vi "ELait03_CriticalValue.vi"(11 "DriverConnect":T1) -> (3 "output string":string)   [LabVIEW 2018]
uses:
  MOKO_LabViewLibrary/MokoLowLevel/MokoLowLovelControl/MLLC_ConnectCluster.ctl
  MOKO_LabViewLibrary/MokoLowLevel/MokoLowLovelControl/MLLC_InterfaceType.ctl
  MOKO_LabViewLibrary/MokoLowLevel/MokoLowLovelControl/MLLC_OpenedSession.ctl
  MOKO_LabViewLibrary/MokoLowLevel/MokoLowLovelControl/MLLC_InterfaceSettings.ctl
  MOKO_LabViewLibrary/MokoLowLevel/MokoLowLovelControl/MLLC_InterfaceKind.ctl
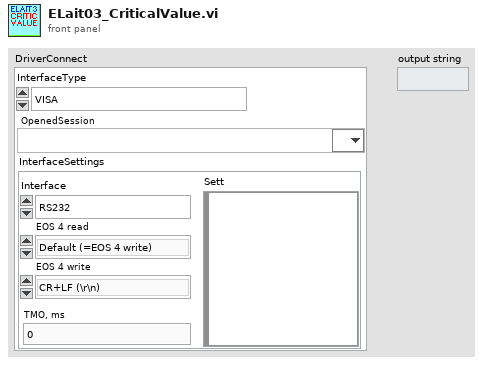
[diagram p1: front panel]
types:
  T1 = typedef "MLLC_ConnectCluster.ctl" = cluster{"InterfaceType":T2, "OpenedSession":T3, "InterfaceSettings":T4}
  T2 = typedef "MLLC_InterfaceType.ctl" = enum16{"VISA", "Prologix USB-GPIB"}
  T3 = typedef "MLLC_OpenedSession.ctl" = refnum<visa-resource-name>
  T4 = typedef "MLLC_InterfaceSettings.ctl" = cluster{"Interface":T5, "EOS 4 read":enum16{"Default (=EOS 4 write)", "CR (\\r)", "LF (\\n)", "None"}, "EOS 4 write":enum16{"CR+LF (\\r\\n)", "CR (\\r)", "LF (\\n)", "None"}, "TMO, ms":i32, "Sett":variant}
  T5 = typedef "MLLC_InterfaceKind.ctl" = enum16{"RS232", "GPIB", "USB", "Ethernet", "another"}
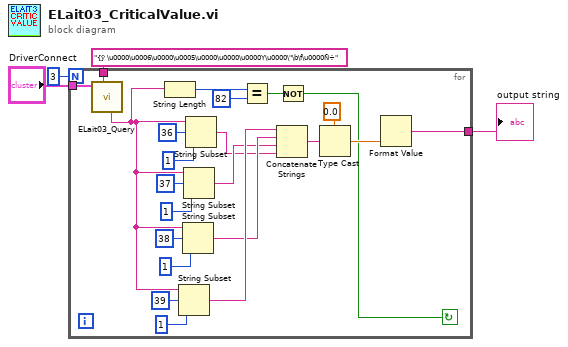
[diagram p0: block diagram]
diagram:
  n1 = for {
    N: 3 -> [_]
    tunnel: "DriverConnect" -> [w12]
    tunnel: "{ÿ \u0000\u0006\u0000\u0005\u0000\u0000\u0000Y\u0000\"\b\f\u0000Ñ÷" -> [w11]
    tunnel: [w10] -> w3
    stop <- w5 continue-if-true
    n2 = call "ELait03_Query.vi"("String"=w11, "DriverConnect in"=w12) -> ("String from device out"=w9:string)  [unwired: 7 in, 2 out]
    n3 = String Length(string=w9) -> (length=w8:i32)
    n4 = String Subset(string=w9, offset (0)=39, length (rest)=1 ("length (rest)")) -> (substring=w17:string)
    n5 = String Subset(string=w9, offset (0)=38, length (rest)=1 ("length (rest)")) -> (substring=w16:string)
    n6 = String Subset(string=w9, offset (0)=37, length (rest)=1 ("length (rest)")) -> (substring=w15:string)
    n7 = String Subset(string=w9, offset (0)=36, length (rest)=1 ("length (rest)")) -> (substring=w14:string)
    n8 = Equal?(x=w8, y=82) -> (x = y?=w6:bool)
    n9 = Concatenate Strings(w17, w16, w15, w14) -> (w13:string)
    n10 = Not(x=w6) -> (.not. x?=w5:bool)
    n11 = Type Cast(type=sgl 0.0, x=w13) -> (*(type *) &x=w18:sgl)
    n12 = Format Value(value (0)=w18) -> (output string=w10:string)  [unwired: 2 in]
  }
  "output string" <- w3
